vi "PicCalib.vi"() -> ()   [LabVIEW 2016]
uses:
  <vilib>/userdefined/High Color/IMAQdx.ctl
  <vilib>/vision/driver/NI_Vision_Acquisition_Software.lvlib
panel:
  out "Angle 2":sgl
  out "Position 2":cluster{"x":sgl, "y":sgl}
  out "Angle":sgl
  out "Position":cluster{"x":sgl, "y":sgl}
  in  "stop":bool
  out "Image":T1(plugin-control)
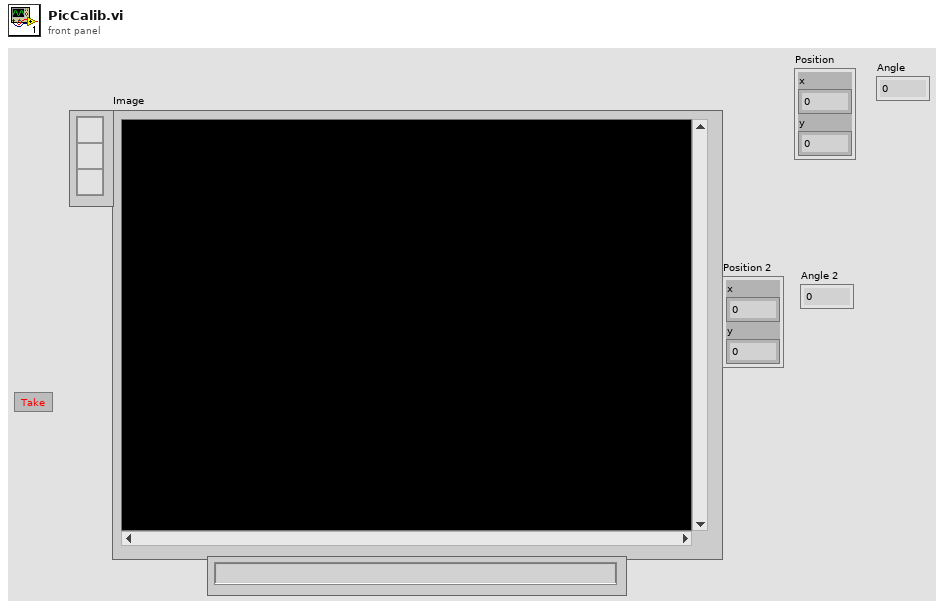
[diagram p1: front panel]
types:
  T1 = typedef "IMAQ Image.ctl" = refnum<image>
  T2 = typedef "IMAQdx.ctl" = refnum<k21>
  T3 = cluster{"Position":cluster{"x":sgl, "y":sgl}, "Angle":sgl, "Scale":sgl, "Score":sgl, "Bounding Box":cluster{"x":sgl, "y":sgl}[]}[]
  T4 = cluster{"Position":cluster{"x":sgl, "y":sgl}, "Angle":sgl, "Scale":sgl, "Score":sgl, "Bounding Box":cluster{"x":sgl, "y":sgl}[]}
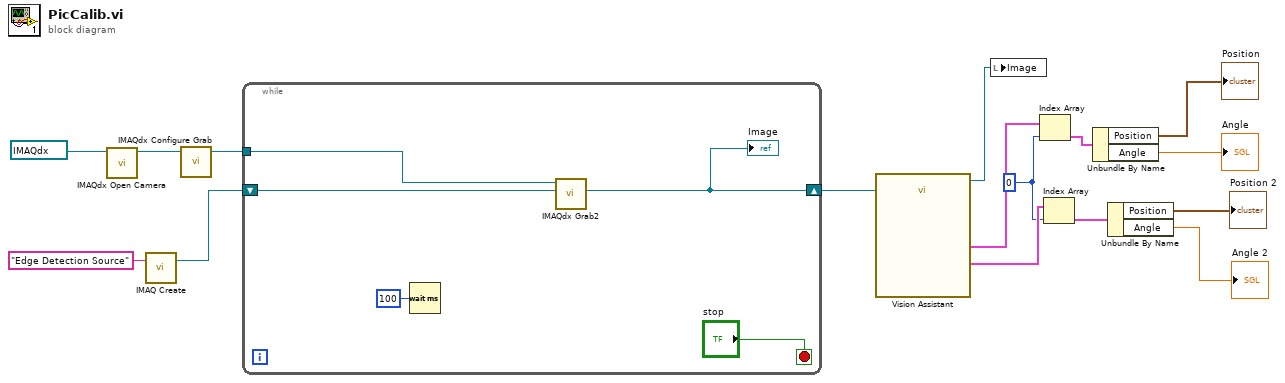
[diagram p0: block diagram]
diagram:
  w8 = 0
  n1 = call <vilib>:"IMAQdx Open Camera.vi"("Session In"=T2 "cam0") -> ("Session Out"=w15:T2)  [unwired: 9 in, 1 out]
  n2 = call "IMAQ Create"("Image Name"="Edge Detection Source") -> ("New Image"=w12:T1)  [unwired: 4 in, 1 out]
  n3 = call <vilib>:"IMAQdx Configure Grab.vi"("Session In"=w15) -> ("Session Out"=w14:T2)  [unwired: 9 in, 1 out]
  n4 = while {
    tunnel: w14 -> [w21]
    shift-right: [w17] -> w11
    shift-left: w12 -> [w20]
    stop <- "stop" stop-if-true
    n5 = Wait (ms)(milliseconds to wait=u32 100) -> ()  [unwired: 1 out]
    n6 = call <vilib>:"IMAQdx Grab2.vi"("Image In"=w20, "Session In"=w21) -> ("Image Out"=w17:T1)  [unwired: 6 in, 3 out]
    "Image" <- w17
  }
  n7 = call "Vision Assistant"("Image In"=w11) -> ("Image Out"=w1:T1, "Matches (Color Pattern Matching 1)"=w10:T3, "Calibrated Matches (Color Pattern Matching 1)"=w9:T3)  [unwired: 22 in, 2 out]
  n8 = local write "Image"(w1) -> ()
  n9 = Index Array(array=w10, index=w8) -> (element=w7:T4)
  n10 = Index Array(array=w9, index=w8) -> (element=w6:T4)
  n11 = Unbundle By Name(w7) -> ("Position"=→"Position":cluster{"x":sgl, "y":sgl}, "Angle"=→"Angle":sgl)
  n12 = Unbundle By Name(w6) -> ("Position"=→"Position 2":cluster{"x":sgl, "y":sgl}, "Angle"=→"Angle 2":sgl)
